vi "GUI.Enable.vi"(7 "VI reference (current VI)":refnum<vi>, 8 "error in (no error)":errorcluster, 10 "Ran?":bool=TRUE, 11 "Array":refnum<vi>[](array[refnum])) -> (0 "error out":errorcluster)   [LabVIEW 2025]
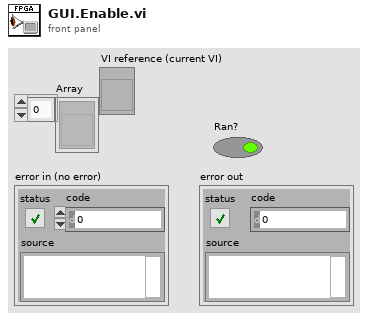
[diagram p1: front panel]
types:
  T1 = enum8{"Enabled", "Disabled", "Disabled and Grayed Out"}
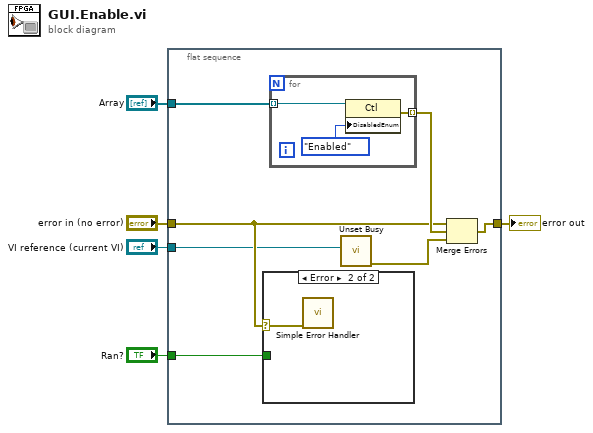
[diagram p0: block diagram]
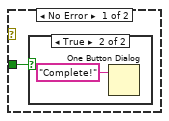
[diagram p2: hidden frame]
diagram:
  n1 = flat-sequence {
    tunnel: "error in (no error)" -> [w9]
    tunnel: "Array" -> [w12]
    tunnel: [w8] -> w5
    tunnel: "VI reference (current VI)" -> [w7]
    tunnel: "Ran?" -> [w6]
    frame #0 {
      n2 = case shown="Error" w9 {
        selector: w9 -> [_ w18]
        tunnel: w6 -> [w16 _]
        frame No Error {
          n3 = case shown="True" w16 {
            frame False {
            }
            frame True {
              n4 = One Button Dialog(message="Complete!") -> ()  [unwired: 1 in, 1 out]
            }
          }
        }
        frame Error {
          n5 = call <vilib>:"Simple Error Handler.vi"("error in (no error)"=w18) -> ()  [unwired: 4 in, 5 out]
        }
      }
      n6 = for {
        tunnel: w12 -> [w15] mode=indexing
        tunnel: [w13] -> w11 mode=indexing
        n7 = property class="Ctl"(reference=w15, "DisabledEnum"=T1."Enabled" ("Disabled")) -> (error out=w13:errorcluster)  [unwired: 1 in, 1 out]
      }
      n8 = call <vilib>:"Unset Busy.vi"("VI reference (current VI)"=w7) -> ("error out"=w10:errorcluster)  [unwired: 10 in]
      n9 = Merge Errors(w9, w11, w10) -> (w8:errorcluster)
    }
  }
  "error out" <- w5
